vi "Get Fixture Object.vi"(8 "error in (no error)":errorcluster, 9 "Routine":T1=enum."Dispense on Plate", 10 "Module In":refnum<class "Module.lvclass">, 11 "Fixture":T2) -> (0 "error out":errorcluster, 2 "Module Out":refnum<class "Module.lvclass">, 3 "Workspace.lvclass":refnum<class "Fixture.lvclass">)   [LabVIEW 2016, in "Fixture.lvclass"]
uses:
  Fixture.lvclass
  Fixture Enum.ctl
  Module/Module.lvclass
  Routine/Routine Enum.ctl
  Carrier Tray/Assembly Tray.lvclass
  D:/LabVIEW/20220413/UCSB-Gantry/V5/Classes/Workspace/Fixture.lvclass
  Component/Component Tray.lvclass
  Pick Up Tool Area/Pick Up Tool Fixture.lvclass
  In Place/Current Position.lvclass
  Carrier Tray/Syringe Space/Syringe Space.lvclass
  Module/Read Instantiated.vi
  Routine/Routine.lvclass
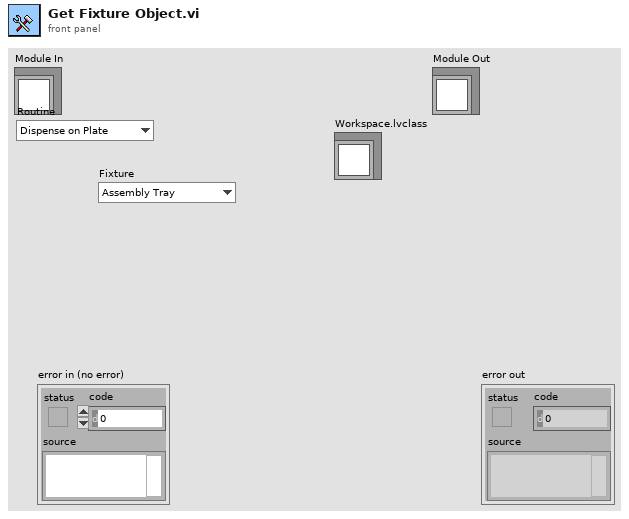
[diagram p1: front panel]
types:
  T1 = typedef "Routine.lvclass/Routine Enum.ctl" = enum16{"Primary Pick Up", "Pick Up All", "Put Down Secondary", "Put Down All", "Release Syringe", "Secondary Pick Up", "Secure Syringe", "Dispense on Plate", "Dispense on Kapton", "Dispense on Sensor", "Dispense on Sensor2"}
  T2 = typedef "Fixture.lvclass/Fixture Enum.ctl" = enum16{"Assembly Tray", "Syringe Space", "Component", "Pick Up Tool", "Current Position"}
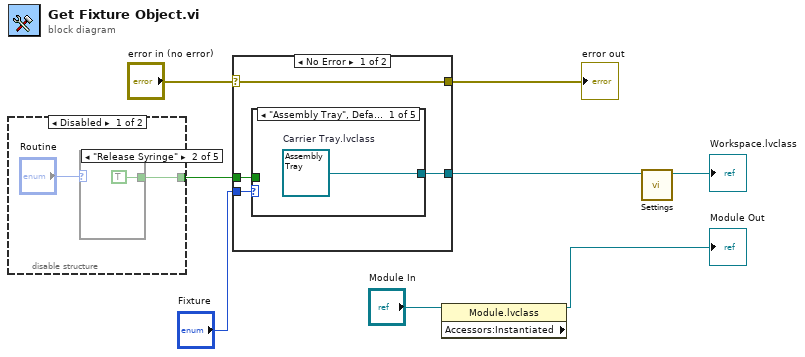
[diagram p0: block diagram]
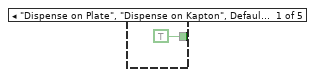
[diagram p2: hidden frame]
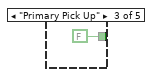
[diagram p3: hidden frame]
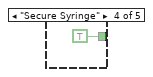
[diagram p4: hidden frame]
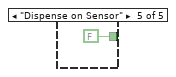
[diagram p5: hidden frame]
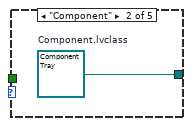
[diagram p7: hidden frame]
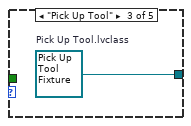
[diagram p8: hidden frame]
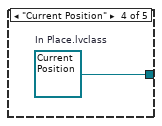
[diagram p9: hidden frame]
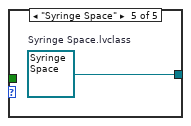
[diagram p10: hidden frame]
diagram:
  n1 = disable-structure shown="Disabled" {
    disable-tunnel: [w9 _] -> w1
    frame Disabled {
      n2 = case shown="\"Release Syringe\"" "Routine" {
        tunnel: [TRUE TRUE FALSE TRUE FALSE] -> w9
        frame "Dispense on Plate", "Dispense on Kapton", Default {
        }
        frame "Release Syringe" {
        }
        frame "Primary Pick Up" {
        }
        frame "Secure Syringe" {
        }
        frame "Dispense on Sensor" {
        }
      }
    }
    frame Enabled {
    }
  }
  n3 = case shown="No Error" "error in (no error)" {
    selector: "error in (no error)" -> [w17 w25]
    tunnel: [w17 w25] -> w7
    tunnel: "Fixture" -> [w19 _]
    tunnel: [w18 _] -> w5
    tunnel: w1 -> [w16 _]
    frame No Error {
      n4 = case shown="\"Assembly Tray\", Default" w19 {
        tunnel: [w20 w21 w22 w23 w24] -> w18
        tunnel: w16 -> [_ _ _ _ _]
        frame "Assembly Tray", Default {
          w20 = refnum<class "Assembly Tray.lvclass"> refnum  # Carrier Tray.lvclass
        }
        frame "Component" {
          w21 = refnum<class "Component Tray.lvclass"> refnum  # Component.lvclass
        }
        frame "Pick Up Tool" {
          w22 = refnum<class "Pick Up Tool Fixture.lvclass"> refnum  # Pick Up Tool.lvclass
        }
        frame "Current Position" {
          w23 = refnum<class "Current Position.lvclass"> refnum  # In Place.lvclass
        }
        frame "Syringe Space" {
          w24 = refnum<class "Syringe Space.lvclass"> refnum  # Syringe Space.lvclass
        }
      }
    }
    frame Error {
    }
  }
  "error out" <- w7
  n5 = property class="Module.lvclass" props=["Accessors:Instantiated"](reference="Module In") -> (reference out=→"Module Out":refnum<class "Module.lvclass">)  [unwired: 1 in, 2 out]
  n6 = call-dynamic "Settings.vi"("Workspace in"=w5) -> ("Workspace out"=→"Workspace.lvclass":refnum<class "Fixture.lvclass">)  [unwired: 9 in, 1 out]
